vi "Draw Cartesian Axes.vi"(5 "[user-specified font]":T3, 6 "Draw Axes":bool, 7 "desired font(Application)":T2(ring)=enum."Application Font", 8 "grid cosmetics":T1={"line color"=39168, "text color"=65280, "tick length(3)"=3, "crossing axes"=FALSE, "visible grid?"=TRUE}, 9 "axis attributes":T5={"x minimum"=0.0, "x maximum"=0.0, "x log?"=FALSE, "x precision"=1, "x format"=enum."Decimal", "y minimum"=0.0, "y maximum"=0.0, "y log?"=FALSE, "y precision"=1, "y format"=enum."Decimal"} {"x minimum" format="%0.2f"; "x maximum" format="%0.2f"; "y minimum" format="%0.2f"; "y maximum" format="%0.2f"}, 10 "bounding rect":T4, 11 "picture":picture) -> (1 "y scale factors":cluster{"a":dbl, "b":dbl, "log?":bool} {"b" format="%0.2f"; "a" format="%0.2f"}, 2 "x scale factors":cluster{"a":dbl, "b":dbl, "log?":bool} {"b" format="%0.2f"; "a" format="%0.2f"}, 3 "new picture":picture)   [LabVIEW 2018, in "Vector Function Generator.xctl"]
doc: "Original version modified by G. Burnell (g.burnell@leeds.ac.uk) for plotting on black background."
uses:
  Vector Function Generator.xctl
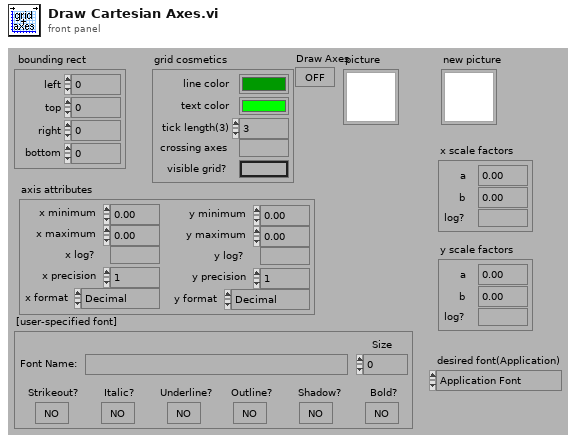
[diagram p1: front panel]
types:
  T1 = cluster{"line color":u32, "text color":u32, "tick length(3)":i16, "crossing axes":bool, "visible grid?":bool}
  T2 = enum16{"User-specified Font", "Application Font", "System Font", "Dialog Font"}
  T3 = cluster{"Font Name:":string, "Size":i16, "Strikeout?":bool, "Italic?":bool, "Underline?":bool, "Outline?":bool, "Shadow?":bool, "Bold?":bool}
  T4 = cluster{"left":i16, "top":i16, "right":i16, "bottom":i16}
  T5 = cluster{"x minimum":dbl, "x maximum":dbl, "x log?":bool, "x precision":u8, "x format":enum8{"Decimal", "Scientific", "Engineering", "Binary", "Octal", "Hex"}, "y minimum":dbl, "y maximum":dbl, "y log?":bool, "y precision":u8, "y format":enum8{"Decimal", "Scientific", "Engineering", "Binary", "Octal", "Hex"}}
  T6 = cluster{"coordinate 1":i16, "value 1":dbl, "coordinate 2":i16, "value 2":dbl, "log?":bool, "fmt and prec":cluster{"format":enum8{"Decimal", "Scientific", "Engineering", "Binary", "Octal", "Hex"}, "precision":u8}}
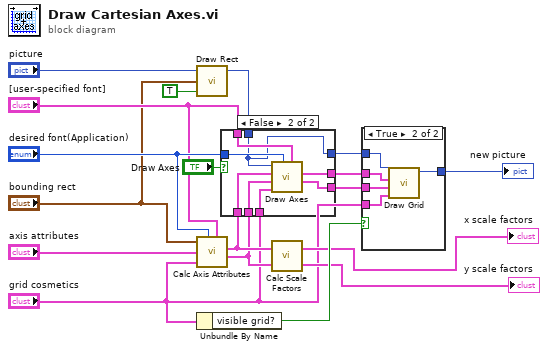
[diagram p0: block diagram]
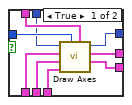
[diagram p2: hidden frame]
diagram:
  n1 = call <vilib>:"Draw Rect.vi"("picture"="picture", "rect"="bounding rect", "fill?(F)"=TRUE) -> ("new picture"=w4:picture)  [unwired: 2 in, 4 out]
  n2 = call <vilib>:"Calc Axis Attributes.vi"("rect"="bounding rect", "desired font(Application)"="desired font(Application)", "xy axis"="axis attributes", "grid cosmetics"="grid cosmetics", "[user-specified font]"="[user-specified font]") -> ("x axis attributes"=w11:T6, "y axis attributes"=w10:T6)  [unwired: 4 out]
  n3 = Unbundle By Name("grid cosmetics") -> ("visible grid?"=w14:bool)
  n4 = case shown="False" "Draw Axes" {
    tunnel: "desired font(Application)" -> [w27 w35]
    tunnel: [w26 w28] -> w17
    tunnel: [w25 w34] -> w16
    tunnel: [w24 w33] -> w15
    tunnel: w11 -> [w23 w32]
    tunnel: w10 -> [w22 w31]
    tunnel: "[user-specified font]" -> [w21 w30]
    tunnel: "grid cosmetics" -> [w20 w29]
    tunnel: w4 -> [w19 w28]
    frame True {
      n5 = call "Draw Axes.vi"("[user-specified font]"=w21, "desired font(Application)"=w27, "grid cosmetics"=w20, "y axis attributes"=w22, "x axis attributes"=w23, "picture"=w19) -> ("y scale specs"=w24:cluster{"coordinate":i16, "label":string}[], "x scale specs"=w25:cluster{"coordinate":i16, "label":string}[], "new picture"=w26:picture)  [unwired: 3 out]
    }
    frame False {
      n6 = call "Draw Axes.vi"("[user-specified font]"=w30, "desired font(Application)"=w35, "grid cosmetics"=w29, "y axis attributes"=w31, "x axis attributes"=w32, "picture"=w28) -> ("y scale specs"=w33:cluster{"coordinate":i16, "label":string}[], "x scale specs"=w34:cluster{"coordinate":i16, "label":string}[])  [unwired: 4 out]
    }
  }
  n7 = call <vilib>:"Calc Scale Factors.vi"("y axis attributes"=w10, "x axis attributes"=w11) -> ("y scale factors"=→"y scale factors":cluster{"a":dbl, "b":dbl, "log?":bool}, "x scale factors"=→"x scale factors":cluster{"a":dbl, "b":dbl, "log?":bool})
  n8 = case shown="True" w14 {
    tunnel: w17 -> [w36 w41]
    tunnel: [w36 w40] -> w12
    tunnel: w16 -> [_ w39]
    tunnel: w15 -> [_ w38]
    tunnel: "grid cosmetics" -> [_ w37]
    frame False {
    }
    frame True {
      n9 = call <vilib>:"Draw Grid.vi"("grid cosmetics"=w37, "y scale specs"=w38, "x scale specs"=w39, "picture"=w41) -> ("new picture"=w40:picture)  [unwired: 5 out]
    }
  }
  "new picture" <- w12
